vi "Serail Modem.vi"(0 "byte count":u32=600, 1 "Write Power Status":bool, 2 "Crew Status":bool[](array[boolean]), 3 "WRITE BUTTON":bool, 5 "error in (no error)":errorcluster, 6 "s? t:f":dbl[](array[numeric]), 8 "piolet/co-p":bool=TRUE) -> (10 "MCC data out":T1 {"TIME" format="%<%H:%M:%S>t"}, 11 "USER STRING":string, 13 "Power  Status":string, 14 "Data out":string, 16 "Data Tx/Rx":string, 17 "Modem Ready Status":bool, 19 "error in (no error) 2":errorcluster)   [LabVIEW 2021]
doc: "This example performs writes and reads on a serial port, as directed by the user. You can press the Write and Read buttons, and change the Read Count, while the example is running.\n\nThe parameters set for the serial port must match the parameters of the connected instrument or device. In this example, the Read Count parameter specifies the number of bytes that the serial port reads. If there were more bytes at the port than the specified number, those bytes would not be read. If there were less bytes at the port than the specified number, you would receive a timeout error.\n\nThis example expands upon the flow control options for XON and XOFF, allowing the user to choose those control characters. Also, the user can enable or disable a termination character. Some devices require a termination character in order to identify the end of command strings. Some devices send a termination character to signify the end of data to be read. This example shows how you can end the Read operation once a termination character is detected in the buffer and/or append a termination character at the end of the Write data."
uses:
  6d023984-3b3b-4ec3-8450-d841155726ca.vi
  <vilib>/Instr/_visa.llb/VISA Configure Serial Port (Instr).vi
  32f44e53-71bb-417d-bfbd-17f234328ae8.vi
panel:
  in  "Enum - Menu":enum16{"Low", "Medium", "High", "Very High"}(ring)
  out "x-y":u32
  out "match substring 2":string
  out "after substring":string
  out "value":sgl[](array[numeric])
  out "before substring":string
  out "substring":string
  out "value 3":i16
  out "value 2":i8
  in  "Battery Status":T2
  out "read buffer":string
  out "length":i32
  out "match substring":string
  in  "stop":bool
  # "Acoustic Telemetry Matsya6000"
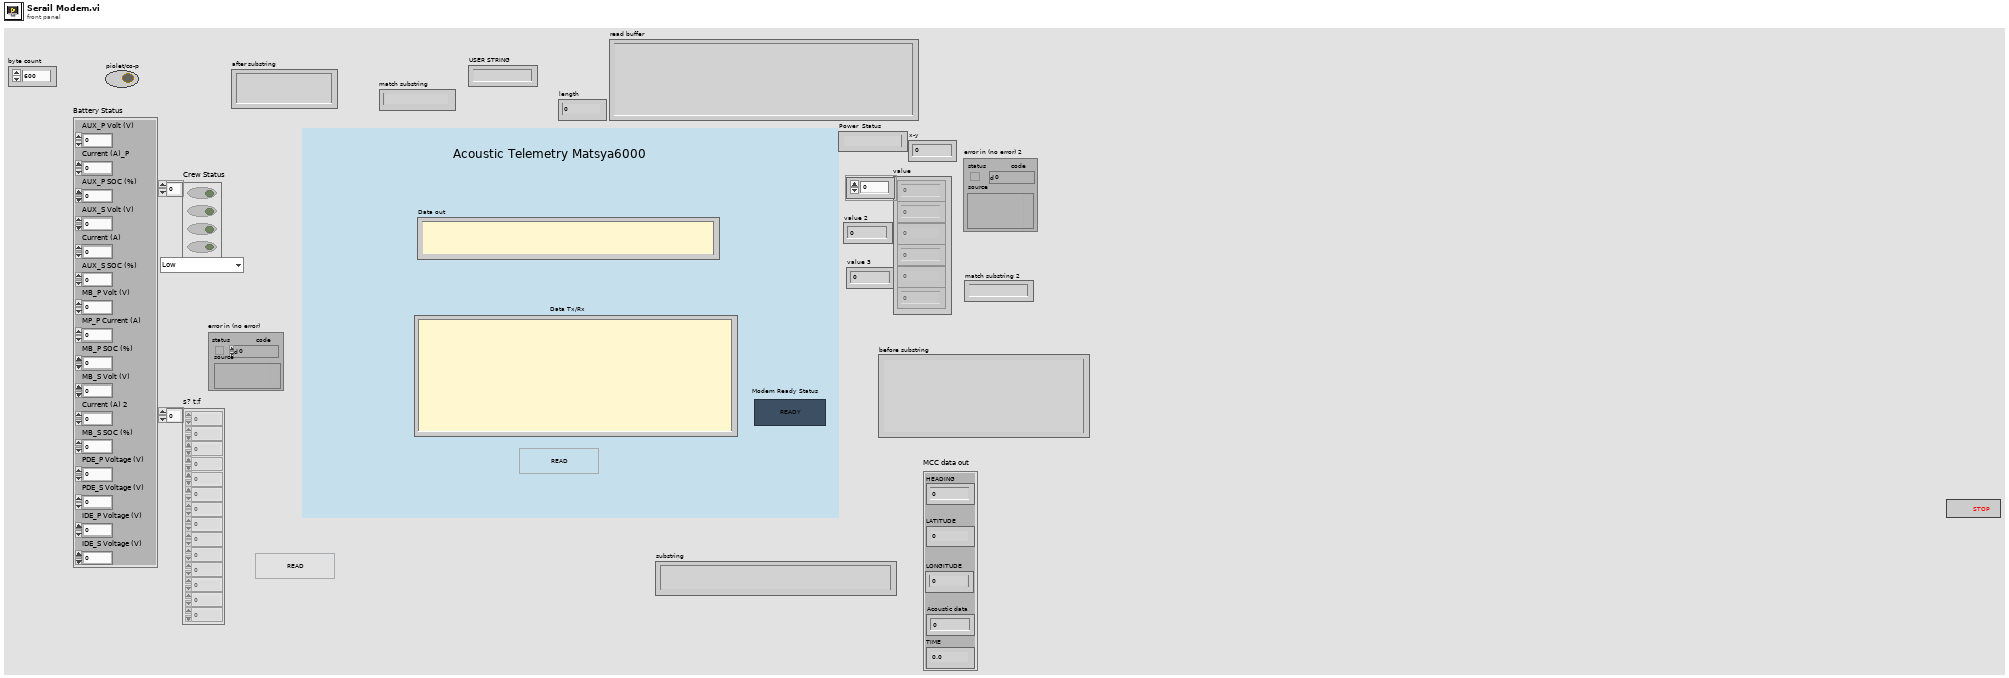
[diagram p1: front panel]
types:
  T1 = cluster{"TIME":sgl, "LATITUDE":sgl, "LONGITUDE":sgl, "HEADING":sgl, "Acoustic data":i32}
  T2 = cluster{"AUX_P Volt (V)":dbl, "Current (A)_P":dbl, "AUX_P SOC (%)":dbl, "AUX_S Volt (V)":dbl, "Current (A)":dbl, "AUX_S SOC (%)":dbl, "MB_P Volt (V)":dbl, "MP_P Current (A)":dbl, "MB_P SOC (%)":dbl, "MB_S Volt (V)":dbl, "Current (A) 2":dbl, "MB_S SOC (%)":dbl, "PDE_P Voltage (V)":dbl, "PDE_S Voltage (V)":dbl, "IDE_P Voltage (V)":dbl, "IDE_S Voltage (V)":dbl}
  T3 = enum16{"read write state", "command mode", "Disable Extended Notification", "bitrate", "initialization", "Int Power Status"}
  T4 = enum16{"read write state", "command mode", "Disable Extended Notification", "bitrate", "initialization"}
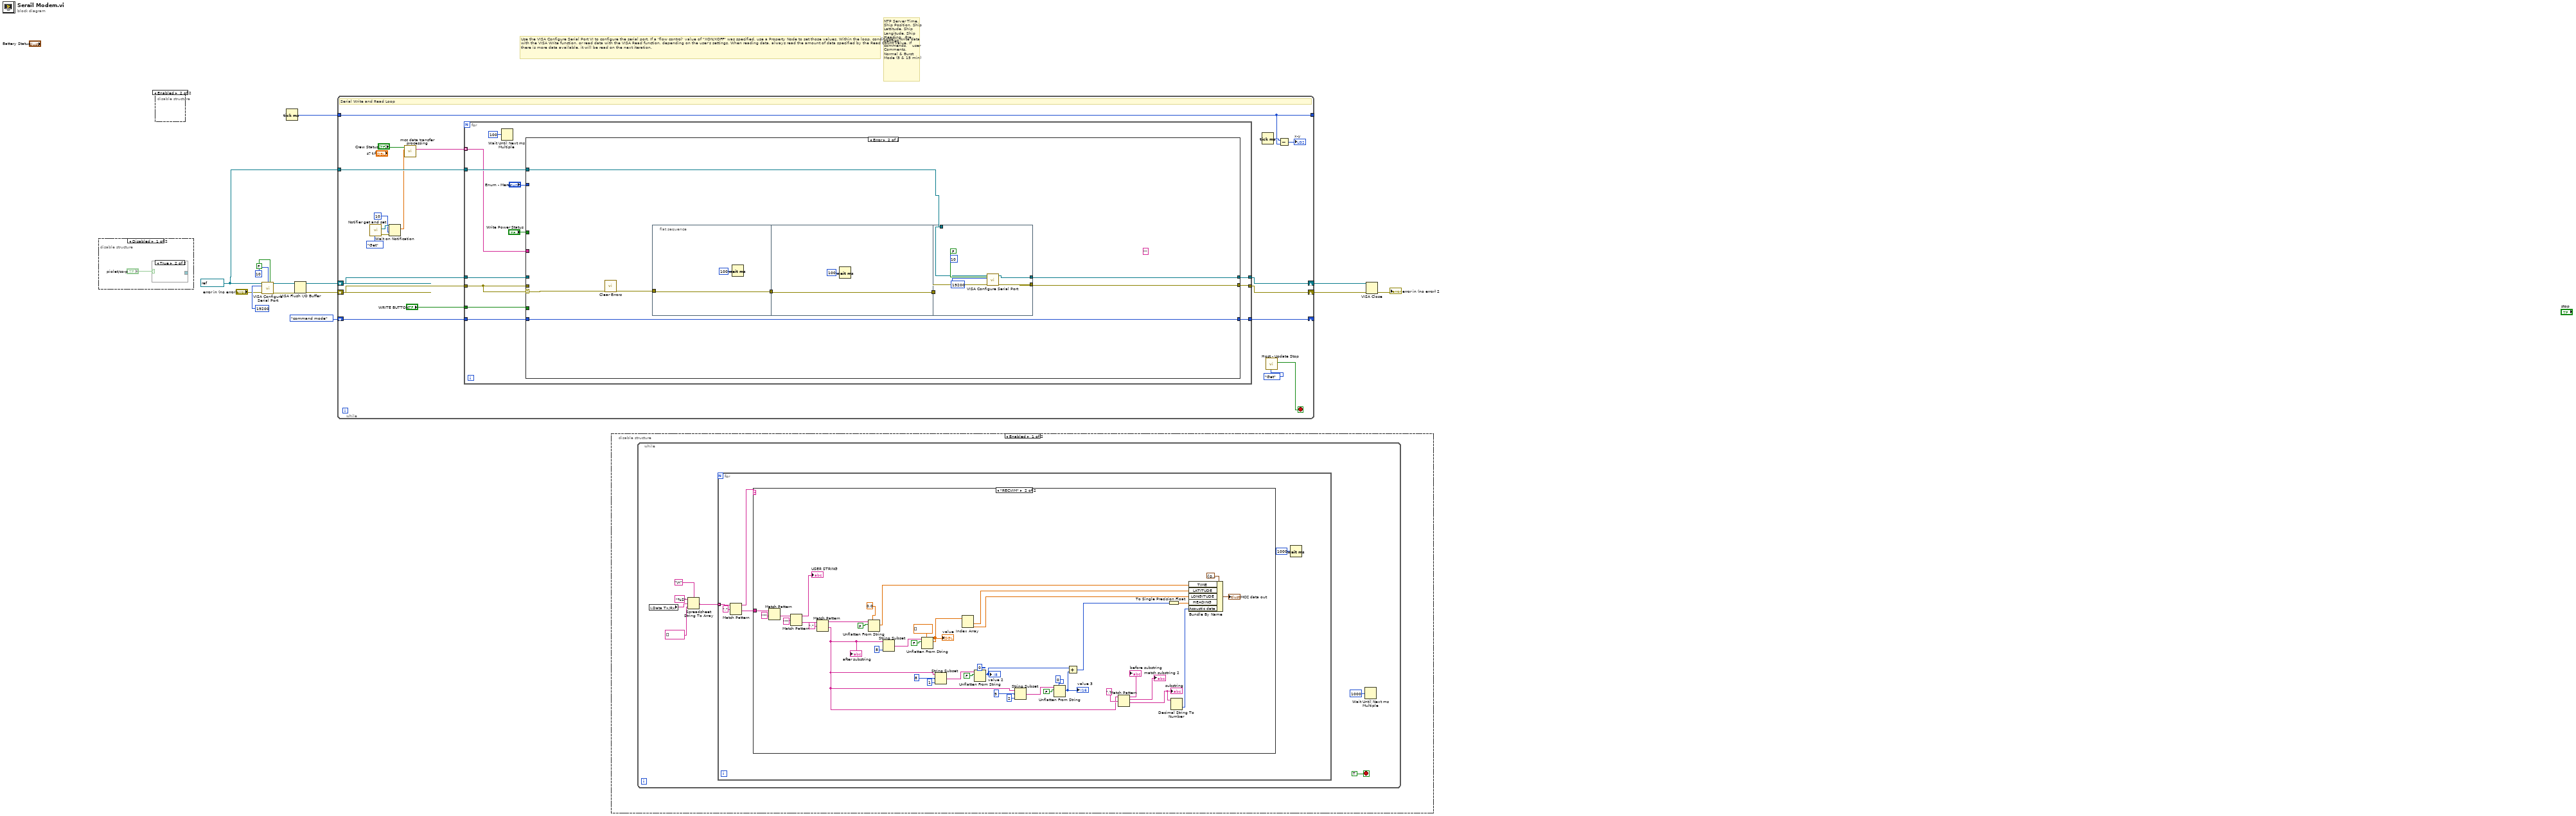
[diagram p0: block diagram]
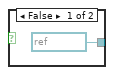
[diagram p4: hidden frame]
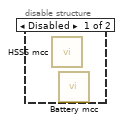
[diagram p6: hidden frame]
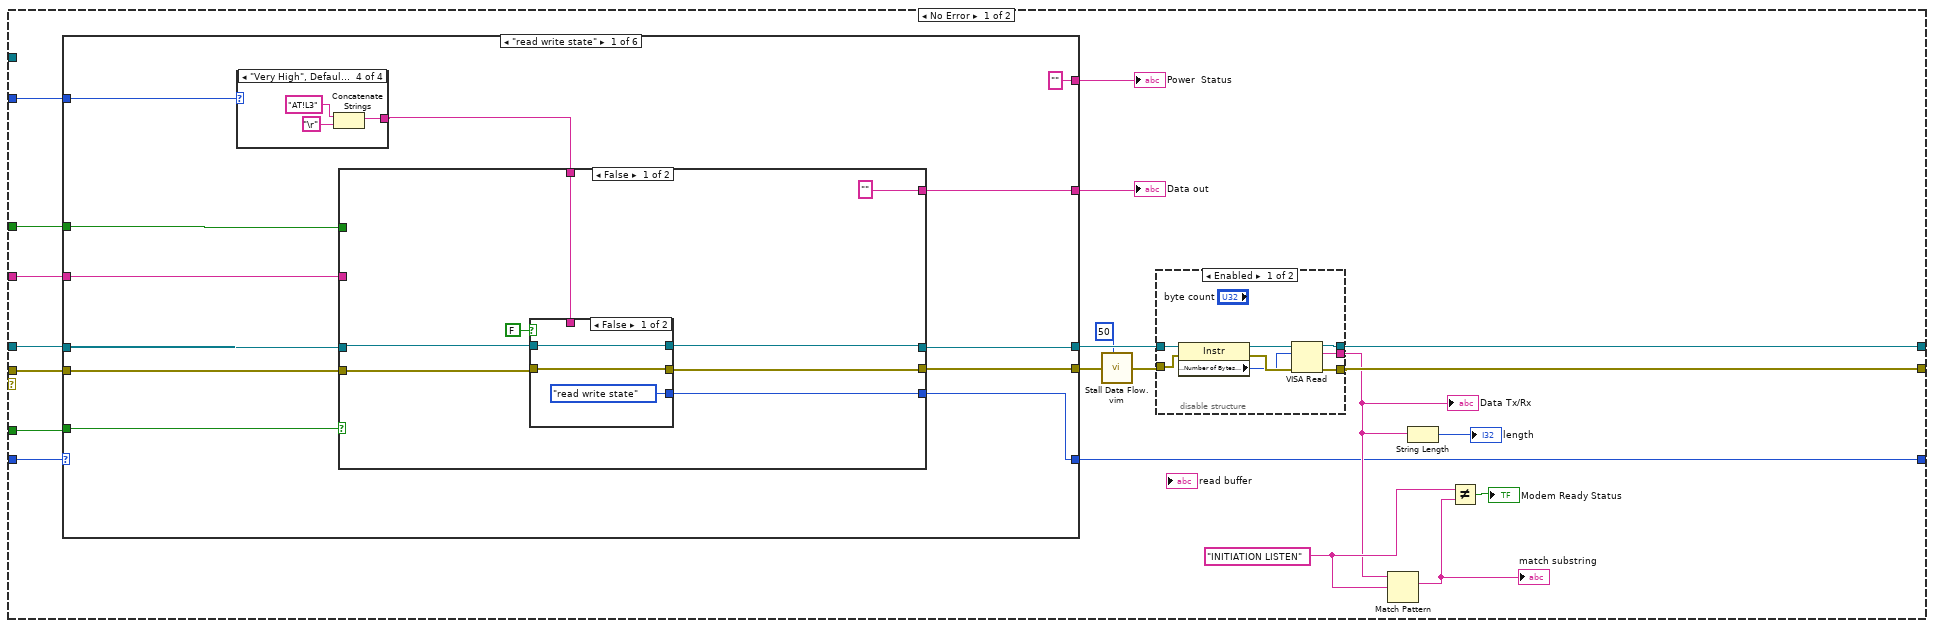
[diagram p7: hidden frame]
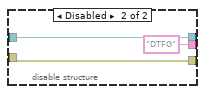
[diagram p8: hidden frame]
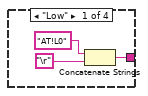
[diagram p9: hidden frame]
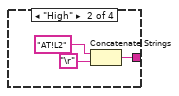
[diagram p10: hidden frame]
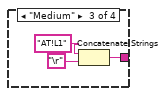
[diagram p11: hidden frame]
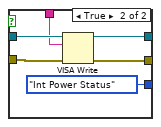
[diagram p12: hidden frame]
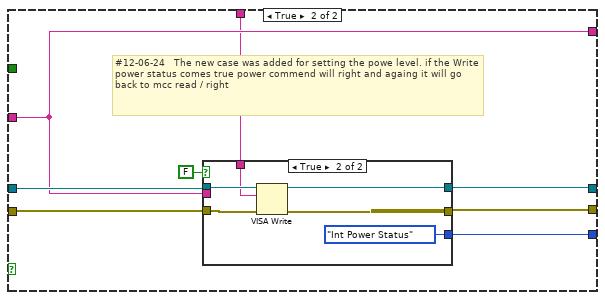
[diagram p13: hidden frame]
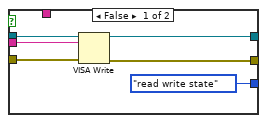
[diagram p14: hidden frame]
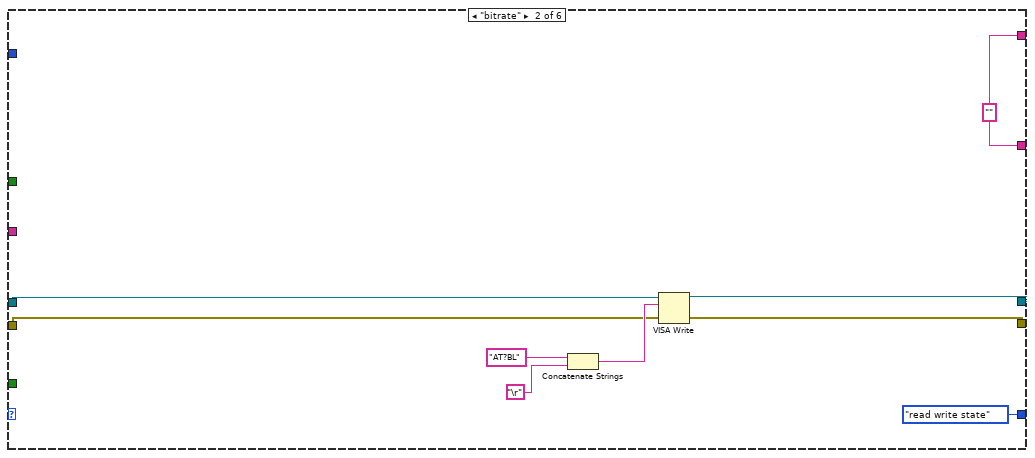
[diagram p15: hidden frame]
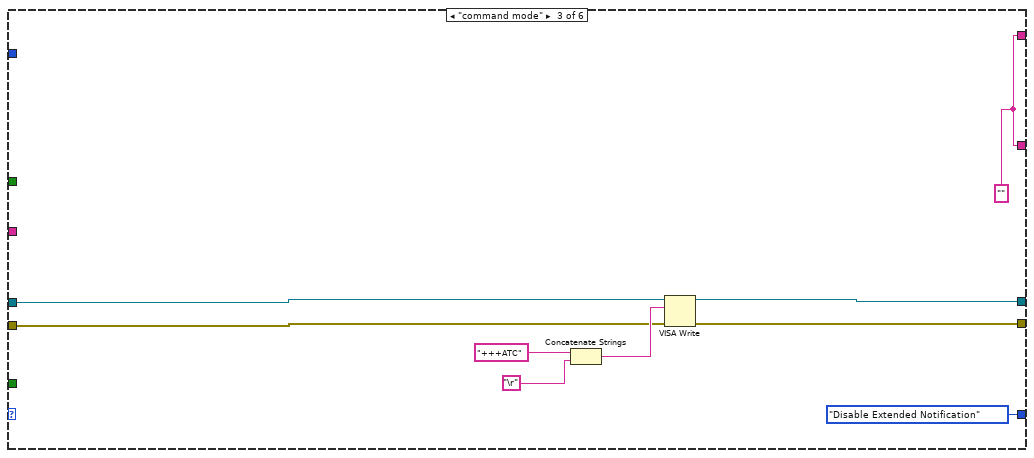
[diagram p16: hidden frame]
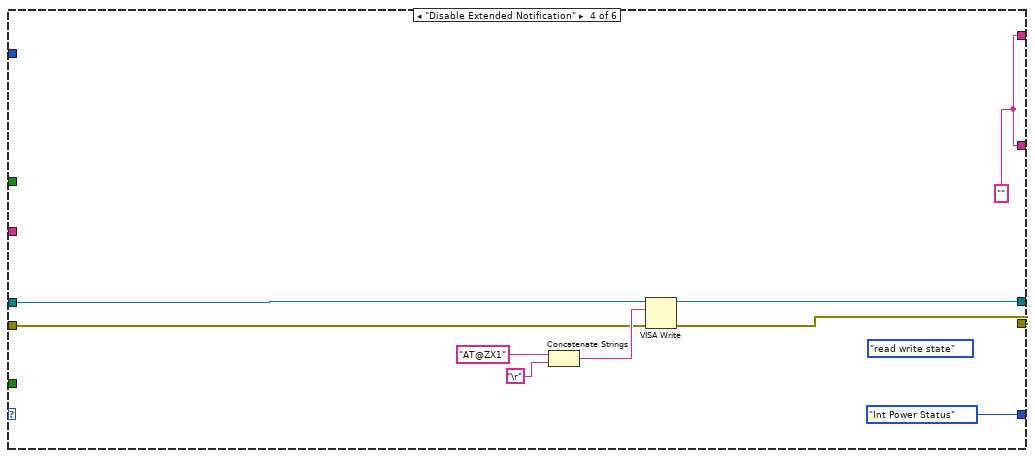
[diagram p17: hidden frame]
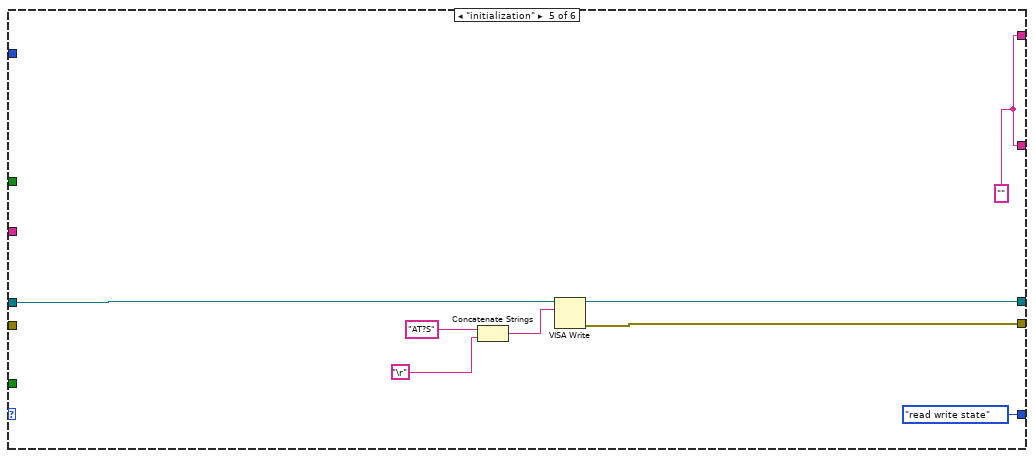
[diagram p18: hidden frame]
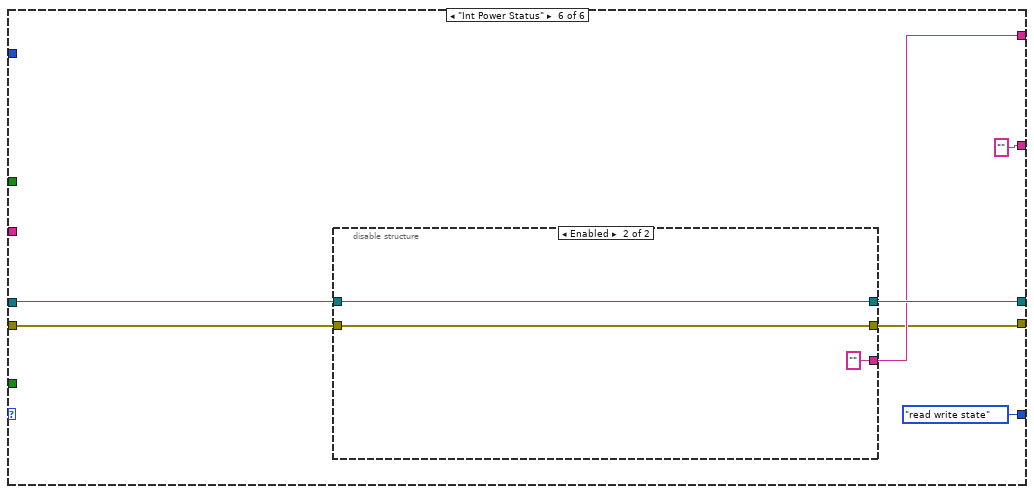
[diagram p19: hidden frame]
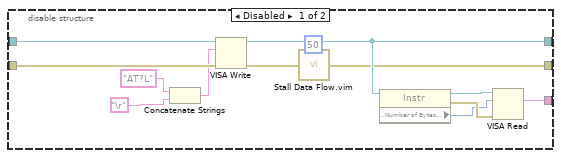
[diagram p20: hidden frame]
diagram:
  w10 = refnum<visa-resource-name> "COM7" ("VISA resource name")
  # "NTP Server Time, Ship Position, Ship Lattitude, Ship Langitude, Ship Heading,  Pre defined commends,    user Comments.  Normal & Burst Mode (5 & 15 min)"
  # "Use the VISA Configure Serial Port VI to configure the serial port. If a 'flow control' value of \"XON/XOFF\" was specified, use a Property Node to set those values. Within the loop, conditionally write data with the VISA Write function, or read data with the VISA Read function, depending on the user's settings. When reading data, always read the amount of data specified by the Read Count value. If there is more data available, it will be read on the next iteration."
  n1 = disable-structure shown="Disabled" {
    frame Disabled {
      n2 = case shown="True" "piolet/co-p" {
        tunnel: [refnum<visa-resource-name> refnum ("VISA resource name") _] -> _
        frame False {
        }
        frame True {
        }
      }
    }
    frame Enabled {
    }
  }
  n3 = disable-structure shown="Enabled" {
    frame Disabled {
      n4 = call "HSSS mcc.vi"() -> ()  [unwired: 12 in]
      n5 = call "Battery mcc.vi"() -> ()  [unwired: 12 in]
    }
    frame Enabled {
    }
  }
  n6 = call-poly "VISA Configure Serial Port"("VISA resource name"=w10, "termination char\n(0xA = '\\n' = LF)"=u8 10 ("termination char\n(0xA = '\\n' = LF)"), "Enable Termination\nChar (T)"=FALSE ("Enable Termination\nChar (T)"), "baud rate (9600)"=u32 19200, "error in (no error)"="error in (no error)") -> ("VISA resource name out"=w5:refnum<visa-resource-name>, "error out"=w6:errorcluster)  [unwired: 9 in]
  n7 = Tick Count (ms)() -> (millisecond timer value=w1:u32)
  n8 = VISA Flush I/O Buffer(VISA resource name=w5, error in (no error)=w6) -> (VISA resource name out=w14:refnum<visa-resource-name>, error out=w13:errorcluster)  [unwired: 1 in]
  n9 = while {
    tunnel: w10 -> [w34]
    shift-right: [w32] -> w3
    shift-left: w14 -> [w36]
    shift-right: [w31] -> w2
    shift-left: w13 -> [w35]
    shift-right: [w30] -> _
    shift-left: T3."command mode" ("Enum") -> [w33]
    tunnel: w1 -> [w24]
    tunnel: [w24] -> _
    stop <- w28 stop-if-true
    # "Serial Write and Read Loop"
    n10 = call "Notifier get and set.vi"("Operation"=enum16{"Init", "Get", "Set"}."Get") -> ("error out"=w19:errorcluster, "notifier out"=w22:refnum<notifier>)  [unwired: 9 in]
    n11 = Wait on Notification(notifier=w22, timeout in ms (-1)=10, error in (no error)=w19) -> (notification=w18:dbl[])  [unwired: 1 in, 3 out]
    n12 = call "mcc data transfer processing.vi"("s? t:f"=w18, "Crew Status"="Crew Status") -> ("appended array"=w26:string[])  [unwired: 3 in, 5 out]
    n13 = for {
      tunnel: w34 -> [w46]
      tunnel: w26 -> [w44] mode=indexing
      tunnel: w33 -> [w45]
      tunnel: [w41] -> w30
      tunnel: w36 -> [w48]
      tunnel: [w43] -> w32
      tunnel: w35 -> [w47]
      tunnel: [w42] -> w31
      tunnel: "WRITE BUTTON" -> [w37]
      n14 = Wait Until Next ms Multiple(millisecond multiple=u32 100) -> ()  [unwired: 1 out]
      n15 = case shown="Error" w47 {
        selector: w47 -> [_ w202]
        tunnel: w48 -> [w69 _]
        tunnel: w47 -> [w68 _]
        tunnel: [w67 w207] -> w43
        tunnel: [w66 w206] -> w42
        tunnel: w46 -> [_ w205]
        tunnel: w37 -> [w62 _]
        tunnel: w45 -> [w58 w200]
        tunnel: w44 -> [w57 _]
        tunnel: [w54 w200] -> w41
        tunnel: "Write Power Status" -> [w52 _]
        tunnel: "Enum - Menu" -> [w49 _]
        frame No Error {
          w65 = "INITIATION LISTEN"
          n16 = case shown="\"read write state\"" w58 {
            tunnel: w69 -> [w92 w145 w157 w166 w174 w182]
            tunnel: w68 -> [w91 w144 w156 w165 _ w183]
            tunnel: [w90 w146 w155 w164 w173 w179] -> w59
            tunnel: [w89 w147 w154 w163 w172 w177] -> w56
            tunnel: w62 -> [w88 _ _ _ _ _]
            tunnel: w57 -> [w87 _ _ _ _ _]
            tunnel: [w86 w142 w151 w160 w169 ""] -> w55
            tunnel: [w81 T3."read write state" ("Enum") T3."Disable Extended Notification" ("Enum") T3."Int Power Status" ("Enum") T3."read write state" ("Enum") T3."read write state" ("Enum")] -> w54
            tunnel: ["" ("read buffer") w142 w151 w160 w169 w178] -> w53
            tunnel: w52 -> [w83 _ _ _ _ _]
            tunnel: w49 -> [w82 _ _ _ _ _]
            frame "read write state" {
              n17 = case shown="\"Very High\", Default" w82 {
                tunnel: [w94 w98 w101 w102] -> w84
                frame "Low" {
                  n18 = Concatenate Strings("AT!L0" ("string"), "\r") -> (w94:string)
                }
                frame "High" {
                  n19 = Concatenate Strings("AT!L2" ("string"), "\r") -> (w98:string)
                }
                frame "Medium" {
                  n20 = Concatenate Strings("AT!L1" ("string"), "\r") -> (w101:string)
                }
                frame "Very High", Default {
                  n21 = Concatenate Strings("AT!L3" ("string"), "\r") -> (w102:string)
                }
              }
              n22 = case shown="False" w88 {
                tunnel: w92 -> [w109 w129]
                tunnel: w91 -> [w111 w128]
                tunnel: [w108 w127] -> w90
                tunnel: [w110 w126] -> w89
                tunnel: w87 -> [_ w125]
                tunnel: ["" w125] -> w86
                tunnel: w84 -> [w107 w124]
                tunnel: w83 -> [_ _]
                tunnel: [w105 w122] -> w81
                frame False {
                  n23 = case shown="False" FALSE {
                    tunnel: w109 -> [w115 w118]
                    tunnel: w111 -> [w114 w121]
                    tunnel: [w115 w119] -> w108
                    tunnel: [w114 w120] -> w110
                    tunnel: w107 -> [_ w117]
                    tunnel: [T3."read write state" ("Enum") T3."Int Power Status" ("Enum")] -> w105
                    frame False {
                    }
                    frame True {
                      n24 = VISA Write(VISA resource name=w118, write buffer=w117, error in (no error)=w121) -> (VISA resource name out=w119:refnum<visa-resource-name>, error out=w120:errorcluster)  [unwired: 1 out]
                    }
                  }
                }
                frame True {
                  # "#12-06-24   The new case was added for setting the powe level. if the Write power status comes true power commend will right and againg it will go back to mcc read / right"
                  n25 = case shown="True" FALSE {
                    tunnel: w129 -> [w135 w138]
                    tunnel: w128 -> [w134 w141]
                    tunnel: [w133 w139] -> w127
                    tunnel: [w132 w140] -> w126
                    tunnel: w125 -> [w131 _]
                    tunnel: w124 -> [_ w137]
                    tunnel: [T3."read write state" ("Enum") T3."Int Power Status" ("Enum")] -> w122
                    frame False {
                      n26 = VISA Write(VISA resource name=w135, write buffer=w131, error in (no error)=w134) -> (VISA resource name out=w133:refnum<visa-resource-name>, error out=w132:errorcluster)  [unwired: 1 out]
                    }
                    frame True {
                      n27 = VISA Write(VISA resource name=w138, write buffer=w137, error in (no error)=w141) -> (VISA resource name out=w139:refnum<visa-resource-name>, error out=w140:errorcluster)  [unwired: 1 out]
                    }
                  }
                }
              }
            }
            frame "bitrate" {
              w142 = ""
              n28 = Concatenate Strings("AT?BL" ("string"), "\r") -> (w150:string)
              n29 = VISA Write(VISA resource name=w145, write buffer=w150, error in (no error)=w144) -> (VISA resource name out=w146:refnum<visa-resource-name>, error out=w147:errorcluster)  [unwired: 1 out]
            }
            frame "command mode" {
              w151 = ""
              n30 = Concatenate Strings("+++ATC" ("string"), "\r") -> (w158:string)
              n31 = VISA Write(VISA resource name=w157, write buffer=w158, error in (no error)=w156) -> (VISA resource name out=w155:refnum<visa-resource-name>, error out=w154:errorcluster)  [unwired: 1 out]
            }
            frame "Disable Extended Notification" {
              w160 = ""
              (unwired) T4."read write state" ("Enum")
              n32 = Concatenate Strings("AT@ZX1" ("string"), "\r") -> (w168:string)
              n33 = VISA Write(VISA resource name=w166, write buffer=w168, error in (no error)=w165) -> (VISA resource name out=w164:refnum<visa-resource-name>, error out=w163:errorcluster)  [unwired: 1 out]
            }
            frame "initialization" {
              w169 = ""
              n34 = Concatenate Strings("AT?S" ("string"), "\r") -> (w176:string)
              n35 = VISA Write(VISA resource name=w174, write buffer=w176) -> (VISA resource name out=w173:refnum<visa-resource-name>, error out=w172:errorcluster)  [unwired: 1 in, 1 out]
            }
            frame "Int Power Status" {
              n36 = disable-structure shown="Enabled" {
                disable-tunnel: w183 -> [w196 w198]
                disable-tunnel: w182 -> [w195 w199]
                disable-tunnel: [w189 w199] -> w179
                disable-tunnel: [w187 "" ("read buffer")] -> w178
                disable-tunnel: [w185 w198] -> w177
                frame Disabled {
                  n37 = Concatenate Strings("AT?L" ("write buffer"), "\r") -> (w193:string)
                  n38 = VISA Write(VISA resource name=w195, write buffer=w193, error in (no error)=w196) -> (VISA resource name out=w189:refnum<visa-resource-name>, error out=w186:errorcluster)  [unwired: 1 out]
                  n39 = call "Stall Data Flow.vim"("value in"=w186, "milliseconds to wait"=u32 50) -> ("value out"=w185:errorcluster)  [unwired: 1 out]
                  n40 = property class="Instr"(reference=w189) -> (reference out=w190:refnum<visa-resource-name>, error out=w191:errorcluster, "Serial Settings:Number of Bytes at Serial Port"=w188:u32)  [unwired: 1 in]
                  n41 = VISA Read(VISA resource name=w190, byte count=w188, error in (no error)=w191) -> (read buffer=w187:string)  [unwired: 3 out]
                }
                frame Enabled {
                }
              }
            }
          }
          "Data out" <- w55
          "Power  Status" <- w53
          n42 = call "Stall Data Flow.vim"("value in"=w56, "milliseconds to wait"=u32 50) -> ("value out"=w51:errorcluster)  [unwired: 1 out]
          n43 = disable-structure shown="Enabled" {
            disable-tunnel: [w77 w80] -> w67
            disable-tunnel: [w76 w79] -> w66
            disable-tunnel: [w73 "DTFG" ("Data Tx/Rx")] -> w61
            disable-tunnel: w59 -> [w72 w80]
            disable-tunnel: w51 -> [w71 w79]
            frame Enabled {
              n44 = property class="Instr"(reference=w72, error in=w71) -> (reference out=w75:refnum<visa-resource-name>, error out=w74:errorcluster, "Serial Settings:Number of Bytes at Serial Port"=w70:u32)
              n45 = VISA Read(VISA resource name=w75, byte count=w70, error in (no error)=w74) -> (VISA resource name out=w77:refnum<visa-resource-name>, read buffer=w73:string, error out=w76:errorcluster)  [unwired: 1 out]
            }
            frame Disabled {
            }
          }
          "Data Tx/Rx" <- w61
          n46 = Match Pattern(string=w61, regular expression=w65) -> (match substring=w64:string)  [unwired: 1 in, 3 out]
          "match substring" <- w64
          n47 = String Length(string=w61) -> (length=→"length":i32)
          n48 = Not Equal?(x=w65, y=w64) -> (x != y?=→"Modem Ready Status":bool)
        }
        frame Error {
          (unwired) ""
          n49 = call <vilib>:"Clear Errors.vi"("error in (no error)"=w202) -> ("error out"=w201:errorcluster)  [unwired: 5 in, 1 out]
          n50 = flat-sequence {
            tunnel: [w208] -> w203
            tunnel: w201 -> [w208]
            tunnel: [w210] -> w204
            tunnel: w203 -> [w210]
            tunnel: [w215] -> w207
            tunnel: [w214] -> w206
            tunnel: w205 -> [w213]
            tunnel: w204 -> [w212]
            frame #0 {
              n51 = Wait (ms)(milliseconds to wait=u32 100) -> ()  [unwired: 1 out]
            }
            frame #1 {
              n52 = Wait (ms)(milliseconds to wait=u32 100) -> ()  [unwired: 1 out]
            }
            frame #2 {
              n53 = call-poly "VISA Configure Serial Port"("VISA resource name"=w213, "termination char\n(0xA = '\\n' = LF)"=u8 10 ("termination char\n(0xA = '\\n' = LF)"), "Enable Termination\nChar (T)"=FALSE ("Enable Termination\nChar (T)"), "baud rate (9600)"=u32 19200, "error in (no error)"=w212) -> ("VISA resource name out"=w215:refnum<visa-resource-name>, "error out"=w214:errorcluster)  [unwired: 5 in, 4 out]
            }
          }
        }
      }
    }
    n54 = Tick Count (ms)() -> (millisecond timer value=w25:u32)
    n55 = call "Host - Update Stop.vi"("Operation"=enum16{"Init", "Get", "Set"}."Get") -> ("Stop?"=w28:bool)  [unwired: 9 in, 1 out]
    n56 = Subtract(x=w25, y=w24) -> (x-y=→"x-y":u32)
  }
  n57 = disable-structure shown="Enabled" {
    frame Enabled {
      n58 = while {
        stop <- TRUE stop-if-true
        n59 = local read "Data Tx/Rx"() -> (w225:string)
        n60 = Spreadsheet String To Array(delimiter (Tab)="\n", format string="%S", spreadsheet string=w225, array type (2D Dbl)=string[] []) -> (array=w223:string[])
        n61 = for {
          tunnel: w223 -> [w230] mode=indexing
          n62 = Match Pattern(string=w230, regular expression=",") -> (before substring=w228:string, after substring=w227:string)  [unwired: 1 in, 2 out]
          n63 = case shown="\"RECVIM\"" w228 {
            tunnel: w227 -> [_ w270]
            frame "USBLANGLES", Default {
            }
            frame "RECVIM" {
              n64 = Match Pattern(string=w270, regular expression="*") -> (after substring=w267:string)  [unwired: 1 in, 3 out]
              n65 = Match Pattern(string=w267, regular expression="*") -> (before substring=→"USER STRING":string, after substring=w264:string)  [unwired: 1 in, 2 out]
              n66 = Match Pattern(string=w264, regular expression=",") -> (before substring=w263:string, after substring=w242:string)  [unwired: 1 in, 2 out]
              "after substring" <- w242
              n67 = Unflatten From String(type=sgl 0.0, binary string=w263, data includes array or string size? (T)=FALSE) -> (value=w236:sgl)  [unwired: 2 in, 2 out]
              n68 = String Subset(string=w242, length (rest)=8 ("length (rest)")) -> (substring=w258:string)  [unwired: 1 in]
              n69 = Unflatten From String(type=sgl[] [], binary string=w258, data includes array or string size? (T)=FALSE) -> (value=w256:sgl[])  [unwired: 2 in, 2 out]
              "value" <- w256
              n70 = String Subset(string=w242, offset (0)=8 ("length (rest)"), length (rest)=1 ("length (rest)")) -> (substring=w254:string)
              n71 = Index Array(array=w256) -> (element #1=w235:sgl, element #2=w234:sgl)  [unwired: 2 in]
              n72 = Unflatten From String(type=i8 0, binary string=w254, data includes array or string size? (T)=FALSE) -> (value=w245:i8)  [unwired: 2 in, 2 out]
              "value 2" <- w245
              n73 = String Subset(string=w242, offset (0)=9 ("length (rest)"), length (rest)=2 ("length (rest)")) -> (substring=w249:string)
              n74 = Unflatten From String(type=i16 0, binary string=w249, data includes array or string size? (T)=FALSE) -> (value=w246:i16)  [unwired: 2 in, 2 out]
              "value 3" <- w246
              n75 = Add(x=w245, y=w246) -> (x+y=w233:i16)
              n76 = Match Pattern(string=w242, regular expression=",") -> (before substring=→"before substring":string, match substring=→"match substring 2":string, after substring=w239:string)  [unwired: 1 in, 1 out]
              "substring" <- w239
              n77 = To Single Precision Float(number=w233) -> (single precision float=w231:sgl)
              n78 = Decimal String To Number(string=w239) -> (number=w232:i32)  [unwired: 2 in, 1 out]
              n79 = Bundle By Name(cluster=T1 {"TIME"=0.0, "LATITUDE"=0.0, "LONGITUDE"=0.0, "HEADING"=0.0, "Acoustic data"=0} ("MCC data out"), "TIME"=w236, "LATITUDE"=w235, "LONGITUDE"=w234, "HEADING"=w231, "Acoustic data"=w232) -> (→"MCC data out":T1)
            }
          }
          n80 = Wait (ms)(milliseconds to wait=u32 1000) -> ()  [unwired: 1 out]
        }
        n81 = Wait Until Next ms Multiple(millisecond multiple=u32 1000) -> ()  [unwired: 1 out]
      }
    }
    frame Disabled {
    }
  }
  n82 = VISA Close(VISA resource name=w3, error in (no error)=w2) -> (error out=→"error in (no error) 2":errorcluster)
